vi "Update(Camera)_v2.vi"(8 "error in (no error)":errorcluster, 10 "Camera_Settings":T2 {"WhiteB." min=2000 max=7500 step=1; "Gain" max=255 step=5; "Exposure" min=0 max=9 step=5; "Focus" step=5}, 11 "Session in":T1) -> (0 "error out":errorcluster, 3 "Session out":T1)   [LabVIEW 2024]
uses:
  Controls/Camera_Settings.ctl
  <vilib>/userDefined/High Color/IMAQdx.ctl
  1c965d0a-2fbf-4a15-954e-c94853878a6e.vi
  5c231780-0e81-4dfd-8826-f815c49f2449.vi
  <resource>/objmgr/imaqdx.rc
  <vilib>/vision/driver/NI_Vision_Acquisition_Software.lvlib
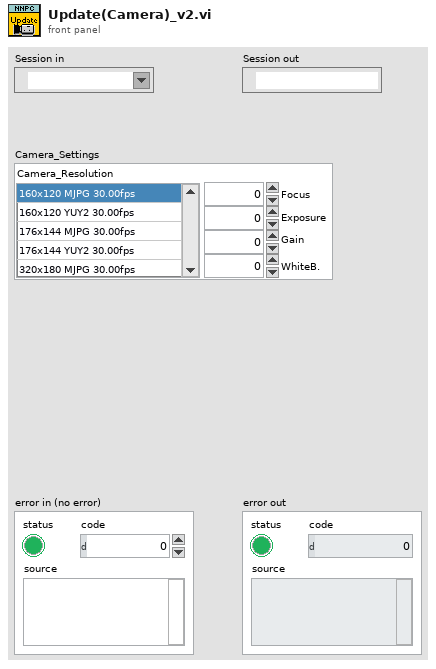
[diagram p1: front panel]
types:
  T1 = typedef "IMAQdx.ctl" = refnum<k21>
  T2 = typedef "Camera_Settings.ctl" = cluster{"Camera_Resolution":i32, "Focus":u8, "Exposure":i32, "Gain":u32, "WhiteB.":i32}
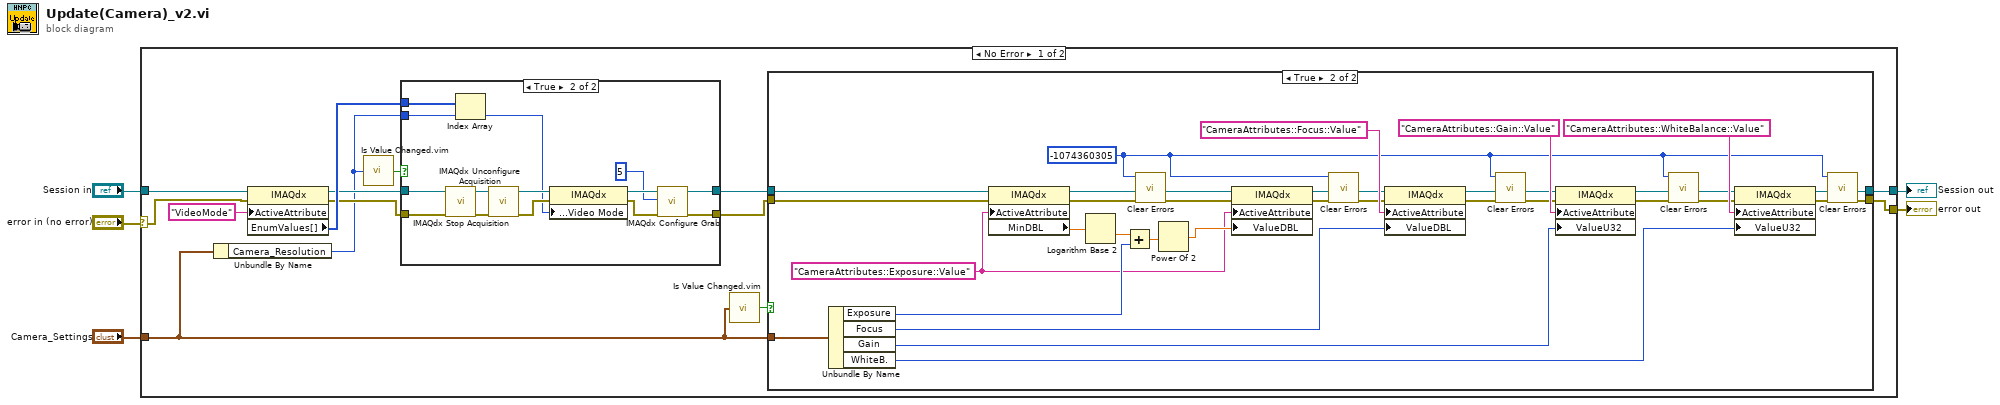
[diagram p0: block diagram]
diagram:
  n1 = case shown="No Error" "error in (no error)" {
    selector: "error in (no error)" -> [w17 w70]
    tunnel: "Session in" -> [w18 w69]
    tunnel: "Camera_Settings" -> [w7 _]
    tunnel: [w10 w69] -> w2
    tunnel: [w9 w70] -> w1
    frame No Error {
      n2 = Unbundle By Name(w7) -> ("Camera_Resolution"=w8:i32)
      n3 = property class="IMAQdx"(reference=w18, error in=w17, "ActiveAttribute"="VideoMode") -> (reference out=w15:T1, error out=w14:errorcluster, "EnumValues[]"=w16:u32[])
      n4 = call "Is Value Changed.vim"("value"=w8) -> ("changed or first call?"=w19:bool)
      n5 = case shown="True" w19 {
        tunnel: [w21 w27] -> w12
        tunnel: [w20 w26] -> w11
        tunnel: w16 -> [_ w35]
        tunnel: w8 -> [_ w34]
        tunnel: w14 -> [w20 w28]
        tunnel: w15 -> [w21 w24]
        frame False {
        }
        frame True {
          n6 = call <vilib>:"IMAQdx Stop Acquisition.vi"("error in"=w28, "Session In"=w24) -> ("error out"=w25:errorcluster, "Session Out"=w23:T1)  [unwired: 8 in]
          n7 = Index Array(array=w35, index=w34) -> (element=w29:u32)
          n8 = call <vilib>:"IMAQdx Unconfigure Acquisition.vi"("error in"=w25, "Session In"=w23) -> ("error out"=w30:errorcluster, "Session Out"=w33:T1)  [unwired: 8 out]
          n9 = property class="IMAQdx"(reference=w33, error in=w30, "Acquisition Attributes:Video Mode"=w29) -> (reference out=w32:T1, error out=w31:errorcluster)
          n10 = call <vilib>:"IMAQdx Configure Grab.vi"("error in"=w31, "Number of Buffers"=u32 5, "Session In"=w32) -> ("error out"=w26:errorcluster, "Session Out"=w27:T1)  [unwired: 1 in, 6 out]
        }
      }
      n11 = call "Is Value Changed.vim"("value"=w7) -> ("changed or first call?"=w6:bool)
      n12 = case shown="True" w6 {
        tunnel: w12 -> [w37 w65]
        tunnel: w11 -> [w36 w64]
        tunnel: [w37 w47] -> w10
        tunnel: [w36 w45] -> w9
        tunnel: w7 -> [_ w39]
        frame False {
        }
        frame True {
          w38 = "CameraAttributes::Exposure::Value" ("ActiveAttribute")
          w40 = -1074360305 ("specific error code to clear (0: all)")
          n13 = Unbundle By Name(w39) -> ("Exposure"=w68:i32, "Focus"=w58:u8, "Gain"=w55:u32, "WhiteB."=w52:i32)
          n14 = property class="IMAQdx"(reference=w65, error in=w64, "ActiveAttribute"=w38) -> (reference out=w51:T1, error out=w62:errorcluster, "MinDBL"=w63:dbl)
          n15 = Logarithm Base 2(1:w63) -> (0:w66:dbl)
          n16 = Add(x=w66, y=w68) -> (x+y=w67:dbl)
          n17 = call <vilib>:"Clear Errors.vi"("error in (no error)"=w62, "specific error code to clear (0: all)"=w40) -> ("error out"=w41:errorcluster)  [unwired: 4 in, 1 out]
          n18 = Power Of 2(x=w67) -> (2^x=w61:dbl)
          n19 = property class="IMAQdx"(reference=w51, error in=w41, "ActiveAttribute"=w38, "ValueDBL"=w61) -> (reference out=w50:T1, error out=w59:errorcluster)
          n20 = call <vilib>:"Clear Errors.vi"("error in (no error)"=w59, "specific error code to clear (0: all)"=w40) -> ("error out"=w42:errorcluster)  [unwired: 4 in, 1 out]
          n21 = property class="IMAQdx"(reference=w50, error in=w42, "ActiveAttribute"="CameraAttributes::Focus::Value", "ValueDBL"=w58) -> (reference out=w49:T1, error out=w56:errorcluster)
          n22 = call <vilib>:"Clear Errors.vi"("error in (no error)"=w56, "specific error code to clear (0: all)"=w40) -> ("error out"=w43:errorcluster)  [unwired: 4 in, 1 out]
          n23 = property class="IMAQdx"(reference=w49, error in=w43, "ActiveAttribute"="CameraAttributes::Gain::Value", "ValueU32"=w55) -> (reference out=w48:T1, error out=w53:errorcluster)
          n24 = call <vilib>:"Clear Errors.vi"("error in (no error)"=w53, "specific error code to clear (0: all)"=w40) -> ("error out"=w44:errorcluster)  [unwired: 4 in, 1 out]
          n25 = property class="IMAQdx"(reference=w48, error in=w44, "ActiveAttribute"="CameraAttributes::WhiteBalance::Value", "ValueU32"=w52) -> (reference out=w47:T1, error out=w46:errorcluster)
          n26 = call <vilib>:"Clear Errors.vi"("error in (no error)"=w46, "specific error code to clear (0: all)"=w40) -> ("error out"=w45:errorcluster)  [unwired: 4 in, 1 out]
        }
      }
    }
    frame Error {
    }
  }
  "Session out" <- w2
  "error out" <- w1
